vi "反控交互.vi"() -> ()   [LabVIEW 2016, in "质控单元V1.lvlib"]
panel:
  in  "启动参数":T1
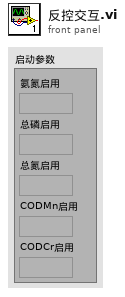
[diagram p1: front panel]
types:
  T1 = cluster{"氨氮启用":bool, "总磷启用":bool, "总氮启用":bool, "CODMn启用":bool, "CODCr启用":bool}
  T2 = typedef "质控单元V1.lvlib/测试流程.ctl" = enum16{"加标回收（启动采配水）", "加标回收（不启动采配水）", "水样测试（启动采配水）", "水样测试（不启动采配水）", "平行样测试（启动采配水）", "平行样测试（不启动采配水）", "集成干预测试"}
  T3 = typedef "质控单元V4.lvlib/数据流类型.ctl" = cluster{"cmd":enum16{"start", "stop"}, "data":variant}
  T4 = typedef "质控slave id.ctl" = enum16{"null", "氨氮", "总磷", "总氮", "CODMn", "CODCr", "氟化物"}
  T5 = cluster{"氨氮静态加标":cluster{"静态加标：":bool, "加标体积":sgl}, "总磷静态加标":cluster{"静态加标：":bool, "加标体积":sgl}, "总氮静态加标":cluster{"静态加标：":bool, "加标体积":sgl}, "CODMn静态加标":cluster{"静态加标：":bool, "加标体积":sgl}, "CODCr静态加标":cluster{"静态加标：":bool, "加标体积":sgl}, "氟化物静态加标":cluster{"静态加标：":bool, "加标体积":sgl}, "挥发酚静态加标":cluster{"静态加标：":bool, "加标体积":sgl}}
  T6 = cluster{"启动参数":cluster{"氨氮启用":bool, "总磷启用":bool, "总氮启用":bool, "CODMn启用":bool, "CODCr启用":bool}, "流程参数":T2}
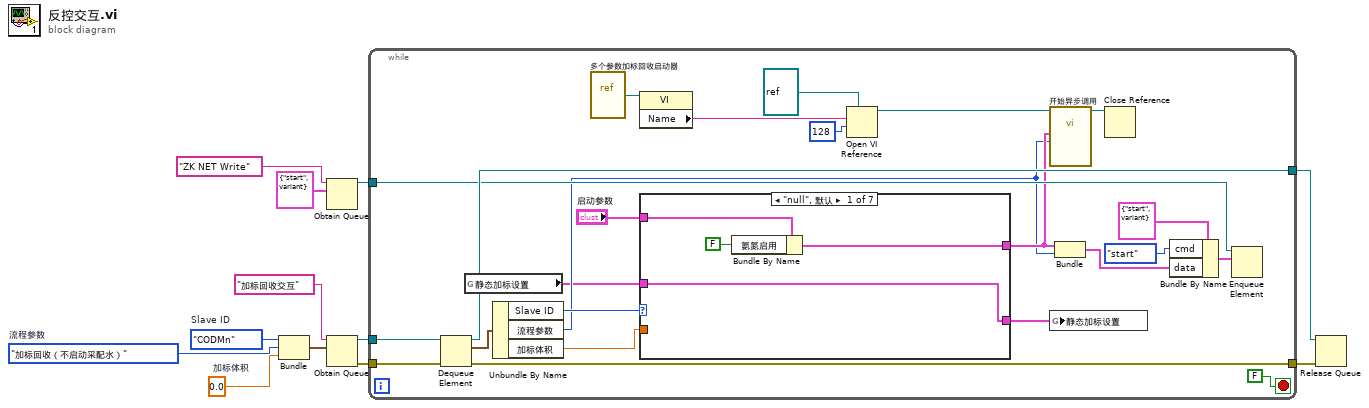
[diagram p0: block diagram]
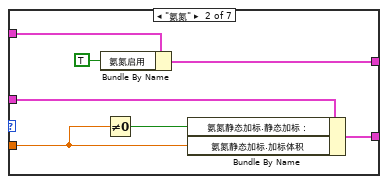
[diagram p2: hidden frame]
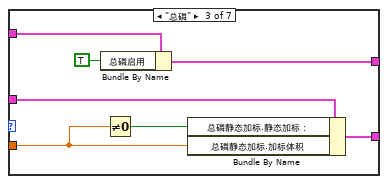
[diagram p3: hidden frame]
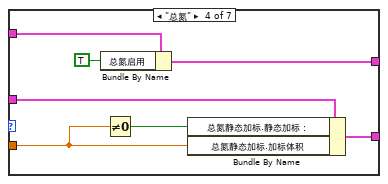
[diagram p4: hidden frame]
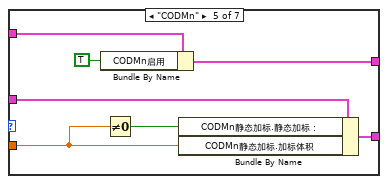
[diagram p5: hidden frame]
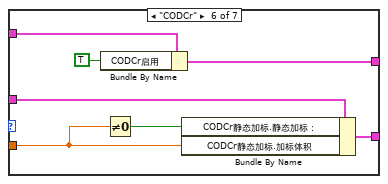
[diagram p6: hidden frame]
diagram:
  w1 = 测试流程."加标回收（不启动采配水）"  # 流程参数
  w2 = sgl 0.0  # 加标体积
  w9 = 质控slave_id."CODMn"  # Slave ID
  n1 = Bundle("Slave ID"=w9, "流程参数"=w1, "加标体积"=w2) -> (w8:cluster{"Slave ID":T4, "流程参数":T2, "加标体积":sgl})  [unwired: 1 in]
  n2 = Obtain Queue(name (unnamed)="ZK NET Write" ("名称（未命名）"), element data type=T3 {"cmd"=enum."start", "data"=variant} ("簇")) -> (queue out=w3:refnum<queue>)  [unwired: 3 in, 2 out]
  n3 = Obtain Queue(name (unnamed)="加标回收交互" ("名称（未命名）"), element data type=w8) -> (queue out=w12:refnum<queue>, error out=w11:errorcluster)  [unwired: 3 in, 1 out]
  n4 = while {
    tunnel: w12 -> [w36]
    tunnel: w11 -> [w35]
    tunnel: [w27] -> w7
    tunnel: [w26] -> w6
    tunnel: w3 -> [w22]
    stop <- FALSE stop-if-true
    n5 = Dequeue Element(queue=w36, error in (no error)=w35) -> (queue out=w27:refnum<queue>, element=w33:cluster{"Slave ID":T4, "流程参数":T2, "加标体积":sgl}, error out=w26:errorcluster)  [unwired: 1 in, 1 out]
    n6 = global read "ZK非断电保存全局变量.vi" "静态加标设置"() -> (w15:T5)
    n7 = Unbundle By Name(w33) -> ("Slave ID"=w28:T4, "流程参数"=w20:T2, "加标体积"=w13:sgl)
    n8 = vi-ref "多个参数加标回收启动器.vi"() -> (w18:refnum<vi>)
    n9 = property class="VI"(reference=w18) -> ("Name"=w32:string)  [unwired: 1 in, 2 out]
    n10 = case shown="\"null\", 默认" w28 {
      tunnel: "启动参数" -> [w39 w47 w53 w61 w68 w75 w77]
      tunnel: [w38 w46 w52 w60 w67 w74 w77] -> w21
      tunnel: w15 -> [w37 w45 w51 w59 w66 w73 w76]
      tunnel: [w37 w43 w50 w57 w64 w71 w76] -> w14
      tunnel: w13 -> [_ w42 w49 w56 w63 w70 _]
      frame "null", Default {
        n11 = Bundle By Name(cluster=w39, "氨氮启用"=FALSE) -> (w38:T1)
      }
      frame "氨氮" {
        n12 = Bundle By Name(cluster=w47, "氨氮启用"=TRUE) -> (w46:T1)
        n13 = Not Equal To 0?(x=w42) -> (x != 0?=w41:bool)
        n14 = Bundle By Name(cluster=w45, "氨氮静态加标.静态加标："=w41, "氨氮静态加标.加标体积"=w42) -> (w43:T5)
      }
      frame "总磷" {
        n15 = Bundle By Name(cluster=w53, "总磷启用"=TRUE ("氨氮启用")) -> (w52:T1)
        n16 = Not Equal To 0?(x=w49) -> (x != 0?=w48:bool)
        n17 = Bundle By Name(cluster=w51, "总磷静态加标.静态加标："=w48, "总磷静态加标.加标体积"=w49) -> (w50:T5)
      }
      frame "总氮" {
        n18 = Bundle By Name(cluster=w61, "总氮启用"=TRUE ("氨氮启用")) -> (w60:T1)
        n19 = Not Equal To 0?(x=w56) -> (x != 0?=w55:bool)
        n20 = Bundle By Name(cluster=w59, "总氮静态加标.静态加标："=w55, "总氮静态加标.加标体积"=w56) -> (w57:T5)
      }
      frame "CODMn" {
        n21 = Bundle By Name(cluster=w68, "CODMn启用"=TRUE ("氨氮启用")) -> (w67:T1)
        n22 = Not Equal To 0?(x=w63) -> (x != 0?=w62:bool)
        n23 = Bundle By Name(cluster=w66, "CODMn静态加标.静态加标："=w62, "CODMn静态加标.加标体积"=w63) -> (w64:T5)
      }
      frame "CODCr" {
        n24 = Bundle By Name(cluster=w75, "CODCr启用"=TRUE ("氨氮启用")) -> (w74:T1)
        n25 = Not Equal To 0?(x=w70) -> (x != 0?=w69:bool)
        n26 = Bundle By Name(cluster=w73, "CODCr静态加标.静态加标："=w69, "CODCr静态加标.加标体积"=w70) -> (w71:T5)
      }
      frame "氟化物" {
      }
    }
    n27 = Open VI Reference(type specifier VI Refnum (for type only)=refnum<vi> refnum, vi path=w32, options=128 ("选项")) -> (vi reference=w30:refnum<vi>)  [unwired: 3 in, 1 out]
    n28 = call-by-ref "开始异步调用"(reference=w30, "流程"=w20, "启用参数选择"=w21) -> (reference out=w29:refnum<vi>)  [unwired: 11 in, 1 out]
    n29 = global write "ZK非断电保存全局变量.vi" "静态加标设置"(w14) -> ()
    n30 = Bundle("启动参数"=w21, "流程参数"=w20) -> (w19:T6)  [unwired: 1 in]
    n31 = Close Reference(reference=w29) -> ()  [unwired: 1 in, 1 out]
    n32 = Bundle By Name(cluster=T3 {"cmd"=enum."start", "data"=variant} ("簇"), "cmd"=enum16{"start", "stop"}."start", "data"=w19) -> (w23:T3)
    n33 = Enqueue Element(queue=w22, element=w23) -> ()  [unwired: 2 in, 3 out]
  }
  n34 = Release Queue(queue=w7, error in (no error)=w6) -> ()  [unwired: 1 in, 3 out]
